vi "telemetryHardpointStatus.vi"(8 "error in (no error)":errorcluster, 11 "Publisher in":refnum<class "Publisher.lvclass">) -> (0 "error out":errorcluster, 3 "Publisher out":refnum<class "Publisher.lvclass">)   [LabVIEW 2016, in "Publisher.lvclass"]
uses:
  Publisher.lvclass
  Publisher.lvclass/Publisher.ctl
  UserEvents/UserEvents.lvclass
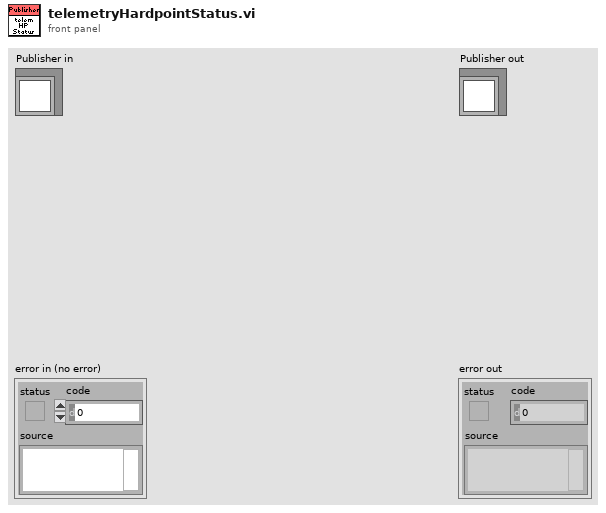
[diagram p1: front panel]
types:
  T1 = typedef "M1M3SupportTopics.lvlib/TelemetryHardpointStatus.ctl" = cluster{"Timestamp":T2, "Mode":u8[], "MajorFault":bool[], "MinorFault":bool[], "FaultOverridden":bool[], "WatchdogReset":bool[], "BrownoutDetected":bool[], "EventTrapReset":bool[], "MotorPowerFault":bool[], "SSRPowerFault":bool[], "AUXPowerFault":bool[], "SMCPowerFault":bool[]}
  T2 = typedef "M1M3SupportTopics.lvlib/Timestamp.ctl" = dbl
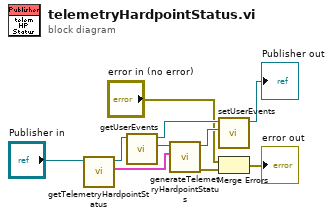
[diagram p0: block diagram]
diagram:
  n1 = call "getTelemetryHardpointStatus.vi"("Publisher in"="Publisher in") -> ("TelemetryHardpointStatus"=w1:T1, "Publisher out"=w9:refnum<class "Publisher.lvclass">)  [unwired: 9 in]
  n2 = call "getUserEvents.vi"("Publisher in"=w9) -> ("UserEvents"=w8:refnum<class "UserEvents.lvclass">, "Publisher out"=w6:refnum<class "Publisher.lvclass">)  [unwired: 9 in]
  n3 = call "generateTelemetryHardpointStatus.vi"("TelemetryHardpointStatus"=w1, "UserEvents in"=w8) -> ("error out"=w4:errorcluster, "UserEvents out"=w7:refnum<class "UserEvents.lvclass">)  [unwired: 8 in]
  n4 = call "setUserEvents.vi"("UserEvents"=w7, "Publisher in"=w6) -> ("Publisher out"=→"Publisher out":refnum<class "Publisher.lvclass">)  [unwired: 9 in]
  n5 = Merge Errors("error in (no error)", w4) -> (→"error out":errorcluster)
